vi "getdojob.vi"(0 "sample port":refnum<visa-resource-name>[](array[refnum]), 2 "sample sn":string[](array[string])) -> (6 "do":dbl[](array[numeric]), 7 "Array":bool[](array[boolean]))   [LabVIEW 2012]
uses:
  globalstatus.vi
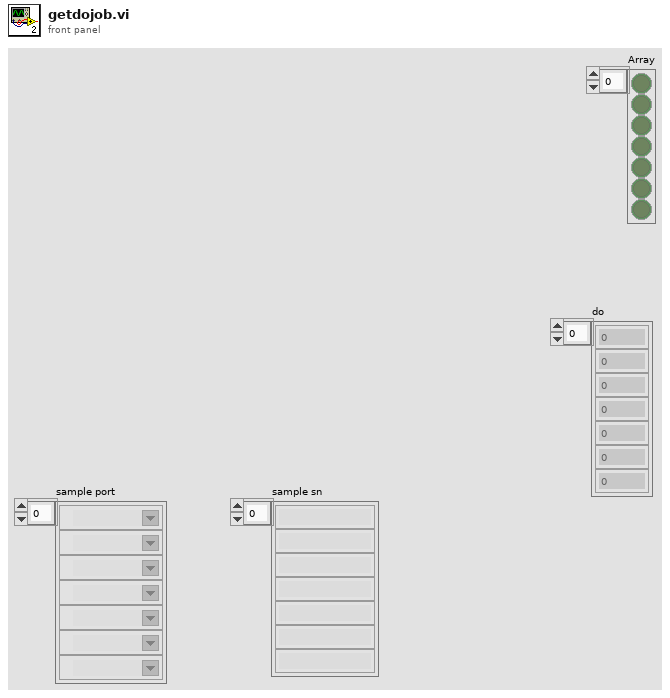
[diagram p1: front panel]
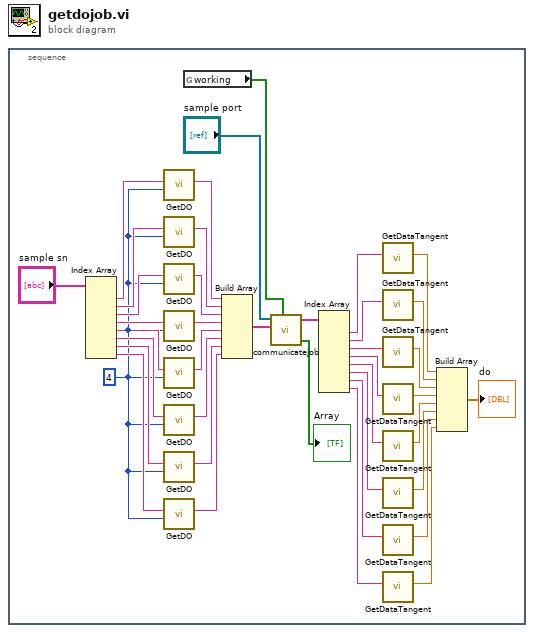
[diagram p0: block diagram]
diagram:
  n1 = stacked-sequence {
    frame #0 {
      w1 = 4
      n2 = Index Array(array="sample sn") -> (element #1=w3:string, element #2=w39:string, element #3=w38:string, element #4=w37:string, element #5=w36:string, element #6=w35:string, element #7=w34:string, element #8=w33:string)  [unwired: 8 in]
      n3 = call "GetDO.vi"("select"=w1, "sn"=w3) -> ("output frame"=w2:string)  [unwired: 9 in]
      n4 = call "GetDO.vi"("select"=w1, "sn"=w39) -> ("output frame"=w30:string)  [unwired: 9 in]
      n5 = call "GetDO.vi"("select"=w1, "sn"=w38) -> ("output frame"=w29:string)  [unwired: 9 in]
      n6 = call "GetDO.vi"("select"=w1, "sn"=w37) -> ("output frame"=w28:string)  [unwired: 9 in]
      n7 = call "GetDO.vi"("select"=w1, "sn"=w36) -> ("output frame"=w27:string)  [unwired: 9 in]
      n8 = call "GetDO.vi"("select"=w1, "sn"=w35) -> ("output frame"=w26:string)  [unwired: 9 in]
      n9 = call "GetDO.vi"("select"=w1, "sn"=w34) -> ("output frame"=w25:string)  [unwired: 9 in]
      n10 = call "GetDO.vi"("select"=w1, "sn"=w33) -> ("output frame"=w24:string)  [unwired: 9 in]
      n11 = global read "globalstatus.vi" "working"() -> (w31:bool[])
      n12 = Build Array(w2, w30, w29, w28, w27, w26, w25, w24) -> (w23:string[])
      n13 = call "communicatejob.vi"("sample port"="sample port", "condition"=w31, "send command"=w23) -> ("receive data"=w21:string[], "receive result"=→"Array":bool[])  [unwired: 2 in, 2 out]
      n14 = Index Array(array=w21) -> (element #1=w20:string, element #2=w19:string, element #3=w18:string, element #4=w17:string, element #5=w16:string, element #6=w15:string, element #7=w14:string, element #8=w13:string)  [unwired: 8 in]
      n15 = call "GetDataTangent.vi"("input data"=w20) -> ("tangent"=w12:dbl)  [unwired: 10 in]
      n16 = call "GetDataTangent.vi"("input data"=w19) -> ("tangent"=w11:dbl)  [unwired: 10 in]
      n17 = call "GetDataTangent.vi"("input data"=w18) -> ("tangent"=w10:dbl)  [unwired: 10 in]
      n18 = call "GetDataTangent.vi"("input data"=w17) -> ("tangent"=w9:dbl)  [unwired: 10 in]
      n19 = call "GetDataTangent.vi"("input data"=w16) -> ("tangent"=w8:dbl)  [unwired: 10 in]
      n20 = call "GetDataTangent.vi"("input data"=w15) -> ("tangent"=w7:dbl)  [unwired: 10 in]
      n21 = call "GetDataTangent.vi"("input data"=w14) -> ("tangent"=w6:dbl)  [unwired: 10 in]
      n22 = call "GetDataTangent.vi"("input data"=w13) -> ("tangent"=w5:dbl)  [unwired: 10 in]
      n23 = Build Array(w12, w11, w10, w9, w8, w7, w6, w5) -> (→"do":dbl[])
    }
  }
